vi "4461 - Create AO waveforms.vi"(8 "error in (no error)":errorcluster, 9 "sampling info":cluster{"Fs":dbl, "#s":dbl}={"Fs"=1000.0, "#s"=1000.0} {"Fs" format="%.2p"}, 10 "reset signal":bool, 11 "AO":T1={"AO amp (V)"=[0.1, 0.09, 0.08, 0.07, 0.06, 0.05, 0.04, 0.03], "AO DC (V)"=[0.0, 0.0, 0.0, 0.0, 0.0, 0.0, 0.0, 0.0], "AO f (Hz)"=[13.0, 13.0, 13.0, 13.0, 13.0, 13.0, 13.0, 13.0], "AO phi (deg)"=[0.0, 0.0, 0.0, 0.0, 0.0, 0.0, 0.0, 0.0], "function"=[enum."Sine Wave", enum."Sine Wave", enum."Sine Wave", enum."Sine Wave", enum."Sine Wave", enum."Sine Wave", enum."Sine Wave", enum."Sine Wave"]} {"AO DC (V)" format="%#_6p"; "AO amp (V)" format="%#_6p"}) -> (0 "error out":errorcluster, 1 "phase out":dbl[](array[numeric]), 2 "AO Array":waveform(dbl)[](array[waveform]), 3 "AO 2":T1={"AO amp (V)"=[0.1, 0.09, 0.08, 0.07, 0.06, 0.05, 0.04, 0.03], "AO DC (V)"=[0.0, 0.0, 0.0, 0.0, 0.0, 0.0, 0.0, 0.0], "AO f (Hz)"=[13.0, 13.0, 13.0, 13.0, 13.0, 13.0, 13.0, 13.0], "AO phi (deg)"=[0.0, 0.0, 0.0, 0.0, 0.0, 0.0, 0.0, 0.0], "function"=[enum."Sine Wave", enum."Sine Wave", enum."Sine Wave", enum."Sine Wave", enum."Sine Wave", enum."Sine Wave", enum."Sine Wave", enum."Sine Wave"]} {"AO DC (V)" format="%#_6p"; "AO amp (V)" format="%#_6p"})   [LabVIEW 2013]
uses:
  <vilib>/Analysis/2dsp.llb/Decimate (single shot).vi
  <vilib>/Analysis/2dsp.llb/Decimate (single shot, DBL).vi
  <vilib>/Utility/error.llb/Error Cluster From Error Code.vi
  <vilib>/measure/NI_MABase.lvlib
panel:
  out "Waveform Graph 2":waveform(dbl)[](graph)=[{"t0"=timestamp(0 s since 1904-01-01), "dt"=4.8828125e-06, "Y"=array[20480 elements]}, {"t0"=timestamp(0 s since 1904-01-01), "dt"=4.8828125e-06, "Y"=array[20480 elements]}, {"t0"=timestamp(0 s since 1904-01-01), "dt"=4.8828125e-06, "Y"=array[20480 elements]}, {"t0"=timestamp(0 s since 1904-01-01), "dt"=4.8828125e-06, "Y"=array[20480 elements]}, {"t0"=timestamp(0 s since 1904-01-01), "dt"=4.8828125e-06, "Y"=array[20480 elements]}, {"t0"=timestamp(0 s since 1904-01-01), "dt"=4.8828125e-06, "Y"=array[20480 elements]}, {"t0"=timestamp(0 s since 1904-01-01), "dt"=4.8828125e-06, "Y"=array[20480 elements]}, {"t0"=timestamp(0 s since 1904-01-01), "dt"=4.8828125e-06, "Y"=array[20480 elements]}]
  out "Numeric":i32
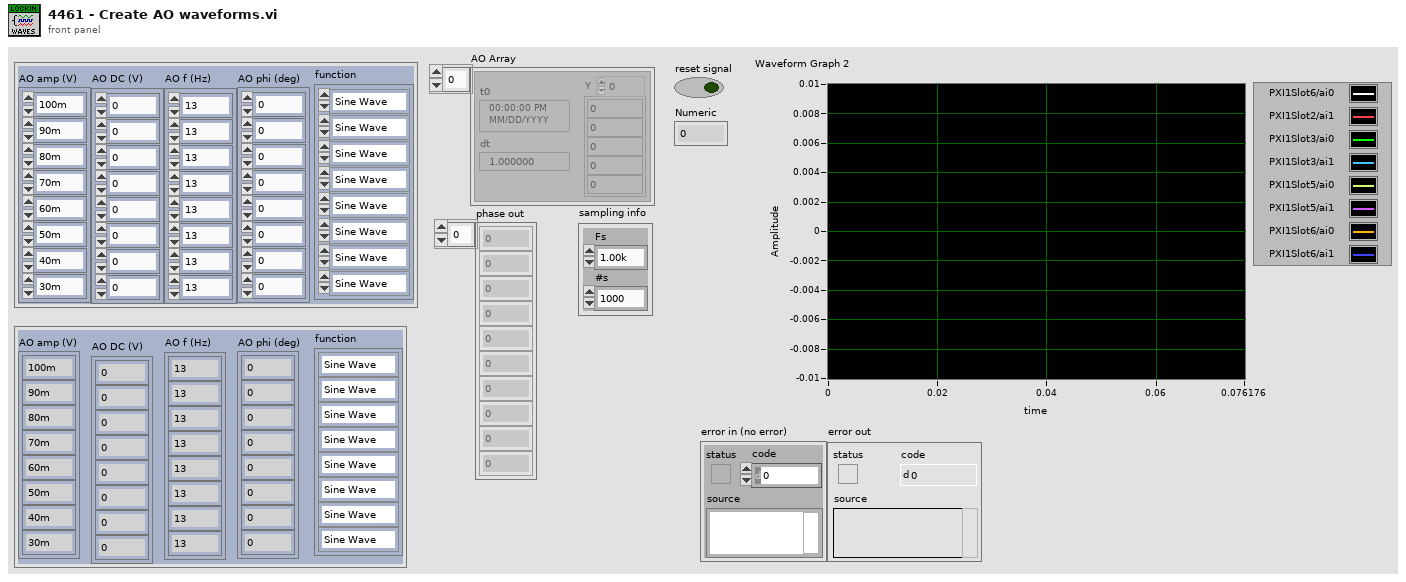
[diagram p1: front panel]
types:
  T1 = cluster{"AO amp (V)":dbl[], "AO DC (V)":dbl[], "AO f (Hz)":dbl[], "AO phi (deg)":dbl[], "function":enum16{"Sine Wave", "Triangle Wave", "Square Wave", "Sawtooth Wave"}[]}
  T2 = enum16{"Sine Wave", "Triangle Wave", "Square Wave", "Sawtooth Wave"}[]
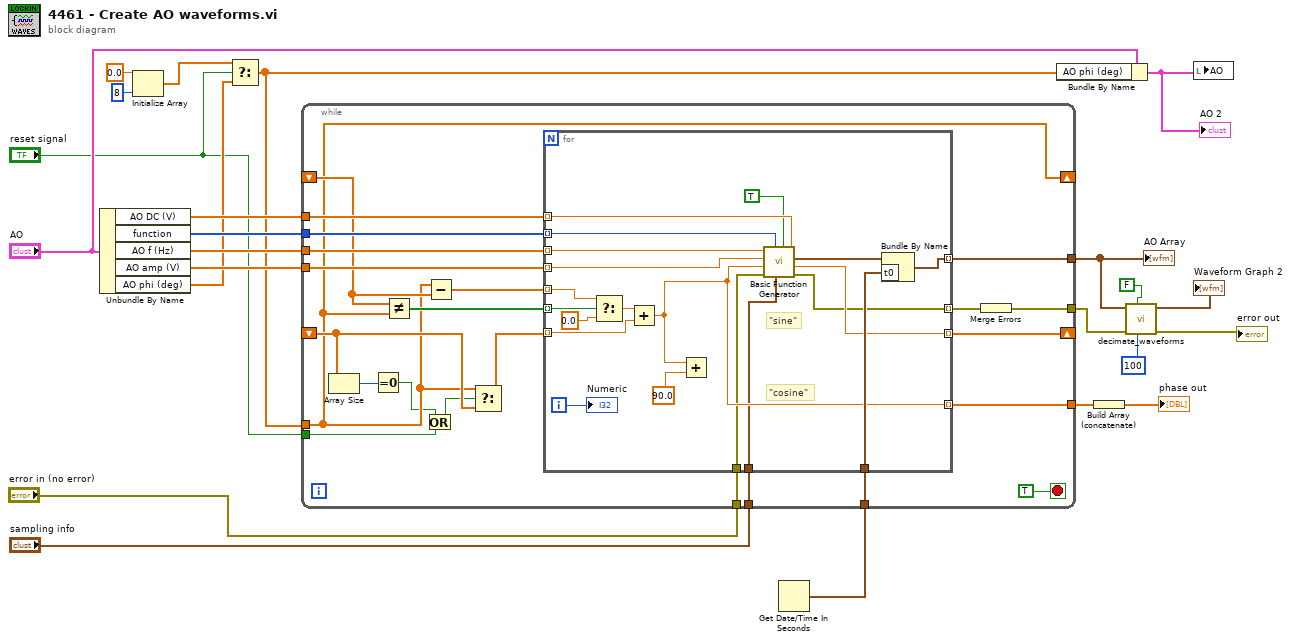
[diagram p0: block diagram]
diagram:
  n1 = Unbundle By Name("AO") -> ("AO DC (V)"=w22:dbl[], "function"=w23:T2, "AO f (Hz)"=w19:dbl[], "AO amp (V)"=w20:dbl[], "AO phi (deg)"=w12:dbl[])
  n2 = Initialize Array(0.0 ("element"), 8 ("dimension size")) -> (w13:dbl[])
  n3 = Select(t=w13, s="reset signal", f=w12) -> (s? t:f=w11:dbl[])
  n4 = Get Date/Time In Seconds() -> (seconds since 1Jan1904=w16:timestamp)
  n5 = while {
    tunnel: w23 -> [w46]
    tunnel: w22 -> [w45]
    tunnel: "sampling info" -> [w44]
    tunnel: [w43] -> w5
    tunnel: w20 -> [w42]
    tunnel: w11 -> [w32]
    tunnel: w19 -> [w41]
    shift-right: [w32] -> _
    shift-left: _ -> [w38]
    shift-right: [w36] -> _
    shift-left: _ -> [w34]
    tunnel: w16 -> [w35]
    tunnel: "reset signal" -> [w29]
    tunnel: [w28] -> w9
    tunnel: "error in (no error)" -> [w26]
    tunnel: [w24] -> w2
    stop <- TRUE stop-if-true
    n6 = Array Size(array=w34) -> (size(s)=w33:i32)
    n7 = Equal To 0?(x=w33) -> (x = 0?=w30:bool)
    n8 = Not Equal?(x=w38, y=w32) -> (x != y?=w39:bool[])
    n9 = Or(x=w30, y=w29) -> (x .or. y?=w31:bool)
    n10 = Subtract(x=w32, y=w38) -> (x-y=w37:dbl[])
    n11 = Select(t=w32, s=w31, f=w34) -> (s? t:f=w27:dbl[])
    n12 = for {
      tunnel: w46 -> [w66] mode=indexing
      tunnel: w41 -> [w65] mode=indexing
      tunnel: w42 -> [w64] mode=indexing
      tunnel: w45 -> [w63] mode=indexing
      tunnel: [w49] -> w43 mode=indexing
      tunnel: w44 -> [w51]
      tunnel: w39 -> [w56] mode=indexing
      tunnel: w37 -> [w58] mode=indexing
      tunnel: [w50] -> w36 mode=indexing
      tunnel: w27 -> [w59] mode=indexing
      tunnel: w35 -> [w55]
      tunnel: [w52] -> w28 mode=indexing
      tunnel: w26 -> [w48]
      tunnel: [w47] -> w25 mode=indexing
      i -> [w54]
      # "\"cosine\""
      # "\"sine\""
      n13 = Select(t=w58, s=w56, f=0.0) -> (s? t:f=w60:dbl)
      n14 = Add(x=w60, y=w59) -> (x+y=w52:dbl)
      n15 = Add(x=w52, y=90.0) -> ()  [unwired: 1 out]
      n16 = call <vilib>:"Basic Function Generator.vi"("offset"=w63, "reset signal"=TRUE, "sampling info"=w51, "signal type"=w66, "error in (no error)"=w48, "phase"=w52, "amplitude"=w64, "frequency"=w65) -> ("error out"=w47:errorcluster, "phase out"=w50:dbl, "signal out"=w62:waveform(dbl))  [unwired: 1 in]
      n17 = Bundle By Name(cluster=w62, "t0"=w55) -> (w49:waveform(dbl))
      "Numeric" <- w54
    }
    n18 = Merge Errors(w25) -> (w24:errorcluster)
  }
  "AO Array" <- w5
  n19 = Bundle By Name(cluster="AO", "AO phi (deg)"=w11) -> (w14:T1)
  "AO 2" <- w14
  n20 = Build Array (concatenate)(w9) -> (→"phase out":dbl[])
  n21 = call "decimate_waveforms.vi"("decimating factor"=100, "averaging"=FALSE, "error in (no error)"=w2, "Input Signal"=w5) -> ("error out"=→"error out":errorcluster, "Decimated Waveforms"=→"Waveform Graph 2":waveform(dbl)[])  [unwired: 6 in]
  n22 = local write "AO"(w14) -> ()
